vi "Prioridade_variaveis_server.vi"(8 "dados_entrada_vindo_client":T1, 11 "padrao_TAGS_prioridade_client":T5) -> (0 "dados_entrada_para_clp_priorizado":T1)   [LabVIEW 2019]
uses:
  padrao_TAGS_prioridades_client.ctl
  padrao_todos_os_dados_SAIDA.ctl
  padrao_UCM.004.EEL.0300_SAIDA.ctl
  padrao_UCM.004.EEL.0200_SAIDA.ctl
  padrao_INTERNO.ctl
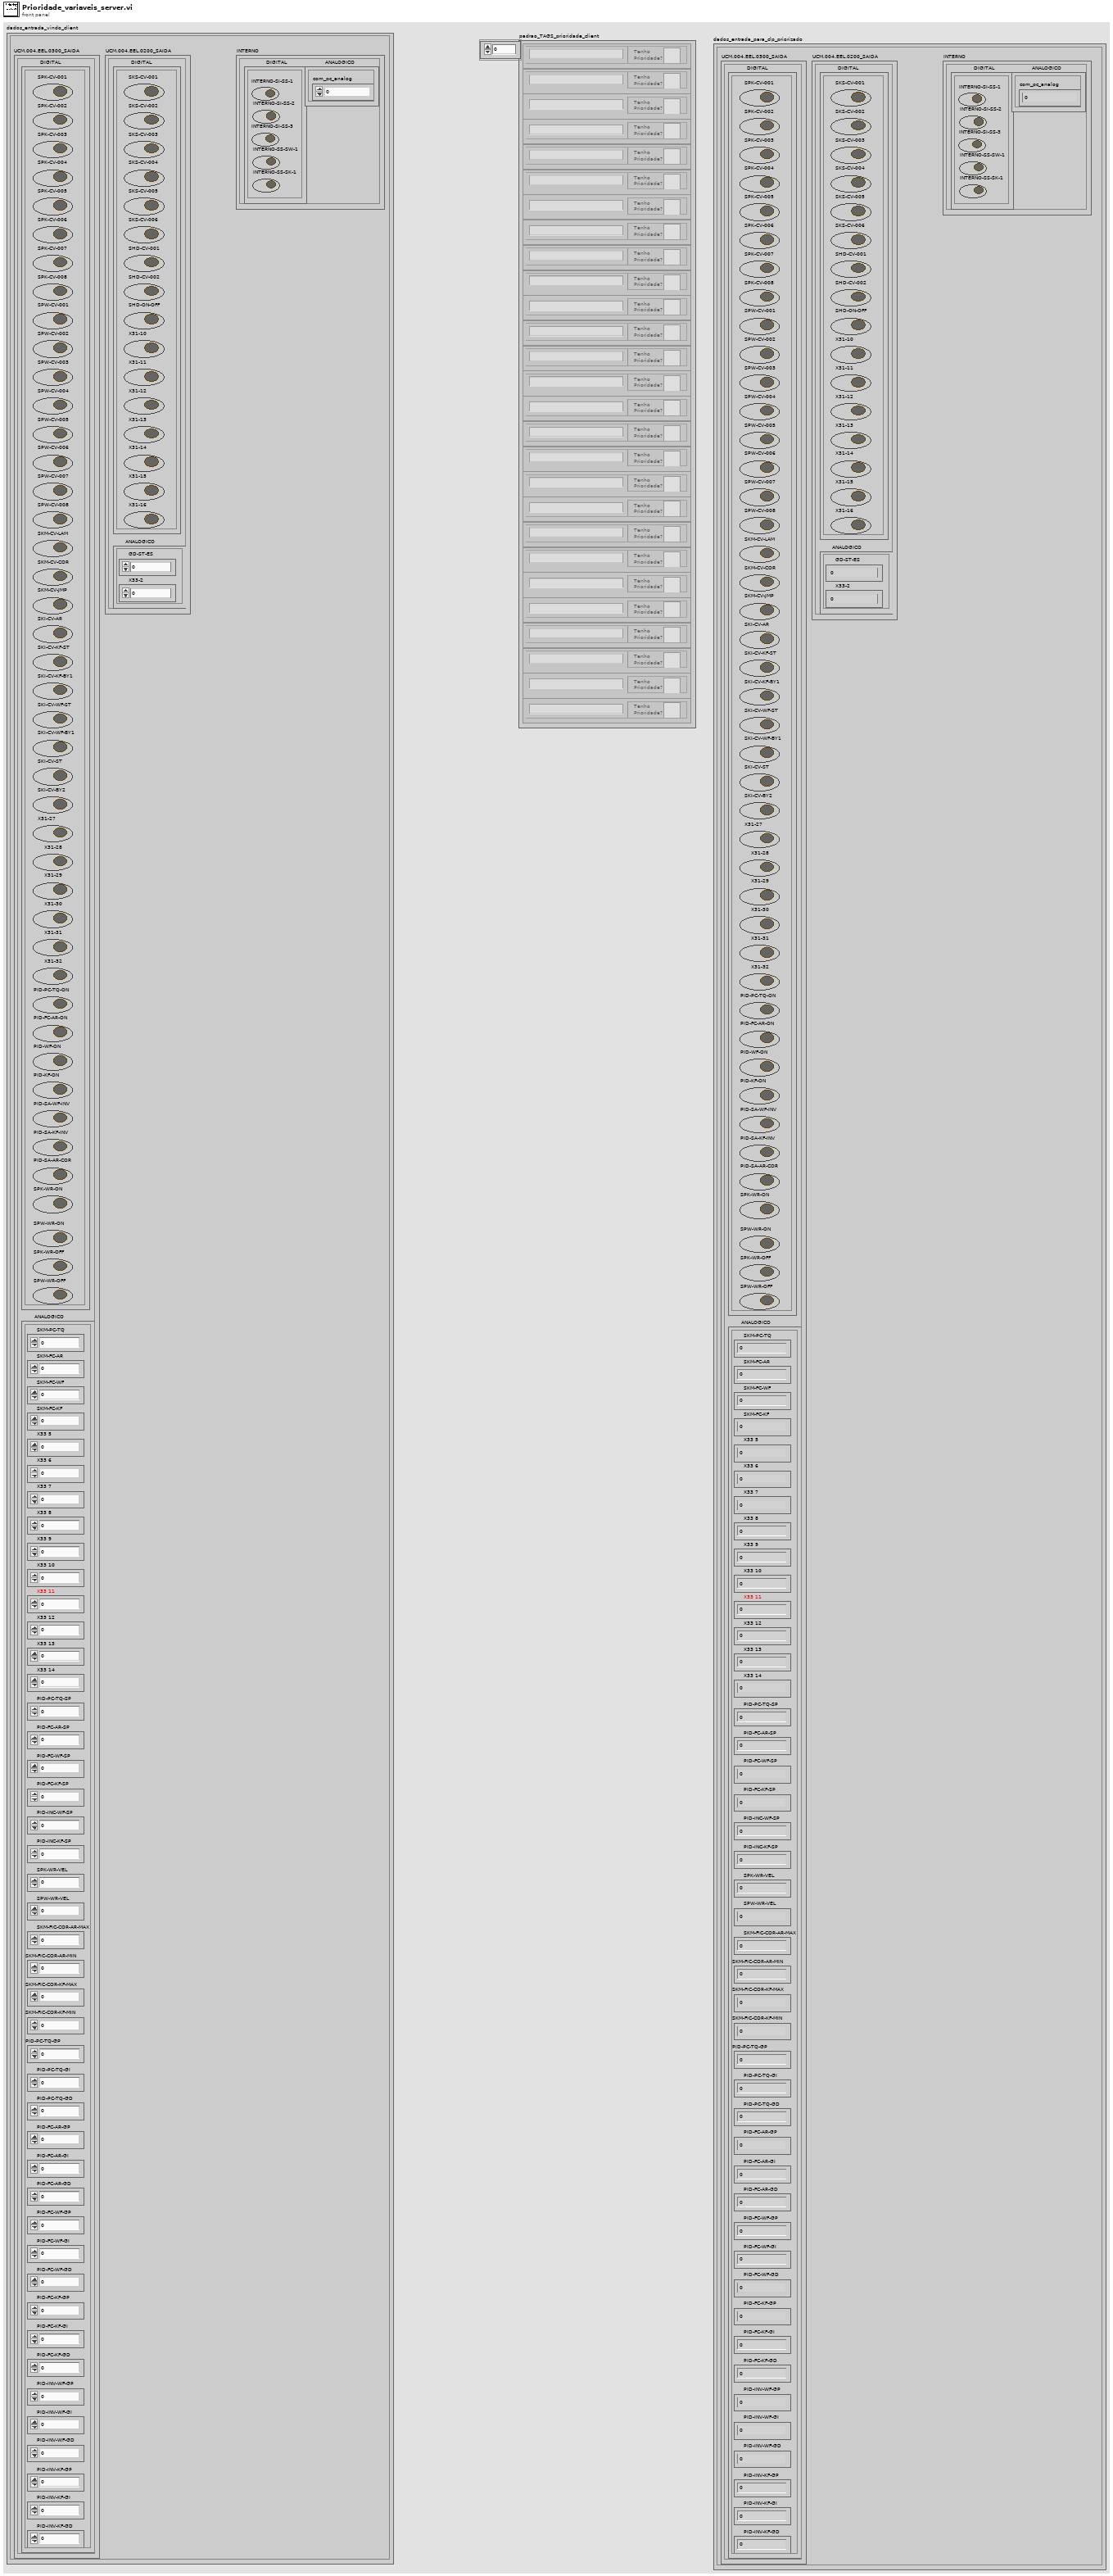
[diagram p1: front panel]
types:
  T1 = typedef "padrao_todos_os_dados_SAIDA.ctl" = cluster{"UCM.004.EEL.0300_SAIDA":T2, "UCM.004.EEL.0200_SAIDA":T3, "INTERNO":T4}
  T2 = typedef "padrao_UCM.004.EEL.0300_SAIDA.ctl" = cluster{"DIGITAL":cluster{"SPK-CV-001":bool, "SPK-CV-002":bool, "SPK-CV-003":bool, "SPK-CV-004":bool, "SPK-CV-005":bool, "SPK-CV-006":bool, "SPK-CV-007":bool, "SPK-CV-008":bool, "SPW-CV-001":bool, "SPW-CV-002":bool, "SPW-CV-003":bool, "SPW-CV-004":bool, "SPW-CV-005":bool, "SPW-CV-006":bool, "SPW-CV-007":bool, "SPW-CV-008":bool, "SKM-CV-LAM":bool, "SKM-CV-COR":bool, "SKM-CV-JMP":bool, "SKI-CV-AR":bool, "SKI-CV-KF-ST":bool, "SKI-CV-KF-BY1":bool, "SKI-CV-WF-ST":bool, "SKI-CV-WF-BY1":bool, "SKI-CV-ST":bool, "SKI-CV-BY2":bool, "X31-27":bool, "X31-28":bool, "X31-29":bool, "X31-30":bool, "X31-31":bool, "X31-32":bool, "PID-PC-TQ-ON":bool, "PID-FC-AR-ON":bool, "PID-WF-ON":bool, "PID-KF-ON":bool, "PID-SA-WF-INV":bool, "PID-SA-KF-INV":bool, "PID-SA-AR-COR":bool, "SPK-WR-ON":bool, "SPW-WR-ON":bool, "SPK-WR-OFF":bool, "SPW-WR-OFF":bool}, "ANALOGICO":cluster{"SKM-PC-TQ":i16, "SKM-FC-AR":i16, "SKM-FC-WF":i16, "SKM-FC-KF":i16, "X33 5":i16, "X33 6":i16, "X33 7":i16, "X33 8":i16, "X33 9":i16, "X33 10":i16, "X33 11":i16, "X33 12":i16, "X33 13":i16, "X33 14":i16, "PID-PC-TQ-SP":i16, "PID-FC-AR-SP":i16, "PID-FC-WF-SP":i16, "PID-FC-KF-SP":i16, "PID-INC-WF-SP":i16, "PID-INC-KF-SP":i16, "SPK-WR-VEL":i32, "SPW-WR-VEL":i32, "SKM-FIC-COR-AR-MAX":dbl, "SKM-FIC-COR-AR-MIN":dbl, "SKM-FIC-COR-KF-MAX":dbl, "SKM-FIC-COR-KF-MIN":dbl, "PID-PC-TQ-GP":dbl, "PID-PC-TQ-GI":dbl, "PID-PC-TQ-GD":dbl, "PID-FC-AR-GP":dbl, "PID-FC-AR-GI":dbl, "PID-FC-AR-GD":dbl, "PID-FC-WF-GP":dbl, "PID-FC-WF-GI":dbl, "PID-FC-WF-GD":dbl, "PID-FC-KF-GP":dbl, "PID-FC-KF-GI":dbl, "PID-FC-KF-GD":dbl, "PID-INV-WF-GP":dbl, "PID-INV-WF-GI":dbl, "PID-INV-WF-GD":dbl, "PID-INV-KF-GP":dbl, "PID-INV-KF-GI":dbl, "PID-INV-KF-GD":dbl}}
  T3 = typedef "padrao_UCM.004.EEL.0200_SAIDA.ctl" = cluster{"DIGITAL":cluster{"SKS-CV-001":bool, "SKS-CV-002":bool, "SKS-CV-003":bool, "SKS-CV-004":bool, "SKS-CV-005":bool, "SKS-CV-006":bool, "SHD-CV-001":bool, "SHD-CV-002":bool, "SHD-ON-OFF":bool, "X31-10":bool, "X31-11":bool, "X31-12":bool, "X31-13":bool, "X31-14":bool, "X31-15":bool, "X31-16":bool}, "ANALOGICO":cluster{"GD-ST-ES":i16, "X33-2":i16}}
  T4 = typedef "padrao_INTERNO.ctl" = cluster{"DIGITAL":cluster{"INTERNO-SI-SS-1":bool, "INTERNO-SI-SS-2":bool, "INTERNO-SI-SS-3":bool, "INTERNO-SS-SW-1":bool, "INTERNO-SS-SK-1":bool}, "ANALOGICO":cluster{"com_pc_analog":dbl}}
  T5 = typedef "padrao_TAGS_prioridades_client.ctl" = cluster{"TAG":string, "Tenho\nPrioridade?":bool}[]
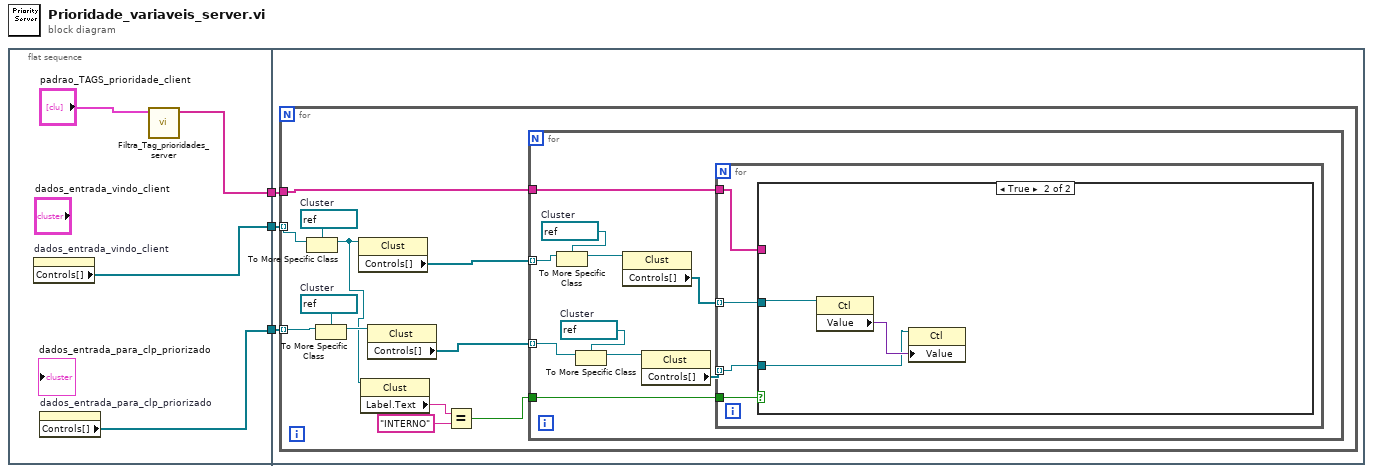
[diagram p0: block diagram]
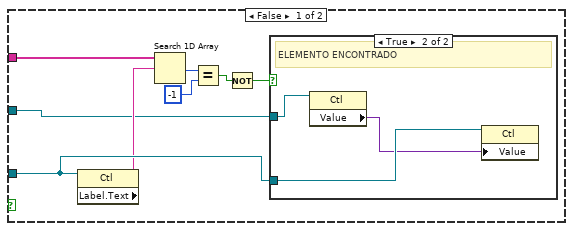
[diagram p2: hidden frame]
diagram:
  n1 = flat-sequence {
    tunnel: [w7] -> w3
    tunnel: [w5] -> w2
    tunnel: [w4] -> w1
    tunnel: w3 -> [w10]
    tunnel: w2 -> [w9]
    tunnel: w1 -> [w8]
    frame #0 {
      n2 = property on="dados_entrada_vindo_client" class="Clust (strict)"() -> ("Controls[]"=w4:refnum<vi>[])  [unwired: 2 in, 2 out]
      n3 = property on="dados_entrada_para_clp_priorizado" class="Clust (strict)"() -> ("Controls[]"=w7:refnum<vi>[])  [unwired: 2 in, 2 out]
      n4 = call "Filtra_Tag_prioridades_server.vi"("padrao_TAGS_prioridade_client"="padrao_TAGS_prioridade_client") -> ("TAGs prioridade"=w5:string[])  [unwired: 10 in]
    }
    frame #1 {
      n5 = for {
        tunnel: w10 -> [w19] mode=indexing
        tunnel: w9 -> [w18]
        tunnel: w8 -> [w16] mode=indexing
        w17 = refnum<vi> refnum  # Cluster
        w22 = refnum<vi> refnum  # Cluster
        n6 = To More Specific Class(target class=w17, reference=w16) -> (specific class reference=w14:refnum<vi>)  [unwired: 1 in, 1 out]
        n7 = To More Specific Class(target class=w22, reference=w19) -> (specific class reference=w20:refnum<vi>)  [unwired: 1 in, 1 out]
        n8 = property on="Property Node" class="Clust"(reference=w14) -> ("Controls[]"=w15:refnum<vi>[])  [unwired: 1 in, 2 out]
        n9 = property class="Clust"(reference=w14) -> ("Label.Text"=w13:string)  [unwired: 1 in, 2 out]
        n10 = property on="Property Node" class="Clust"(reference=w20) -> ("Controls[]"=w21:refnum<vi>[])  [unwired: 1 in, 2 out]
        n11 = Equal?(x=w13, y="INTERNO") -> (x = y?=w11:bool)
        n12 = for {
          tunnel: w21 -> [w31] mode=indexing
          tunnel: w18 -> [w28]
          tunnel: w15 -> [w25] mode=indexing
          tunnel: w11 -> [w23]
          w27 = refnum<vi> refnum  # Cluster
          w30 = refnum<vi> refnum  # Cluster
          n13 = To More Specific Class(target class=w27, reference=w25) -> (specific class reference=w26:refnum<vi>)  [unwired: 1 in, 1 out]
          n14 = To More Specific Class(target class=w30, reference=w31) -> (specific class reference=w32:refnum<vi>)  [unwired: 1 in, 1 out]
          n15 = property on="Property Node" class="Clust"(reference=w26) -> ("Controls[]"=w24:refnum<vi>[])  [unwired: 1 in, 2 out]
          n16 = property on="Property Node" class="Clust"(reference=w32) -> ("Controls[]"=w29:refnum<vi>[])  [unwired: 1 in, 2 out]
          n17 = for {
            tunnel: w29 -> [w36] mode=indexing
            tunnel: w28 -> [w35]
            tunnel: w24 -> [w34] mode=indexing
            tunnel: w23 -> [w33]
            n18 = case shown="True" w33 {
              tunnel: w36 -> [w44 w48]
              tunnel: w35 -> [w43 _]
              tunnel: w34 -> [w37 w49]
              frame False {
                n19 = property class="Ctl"(reference=w44) -> ("Label.Text"=w42:string)  [unwired: 1 in, 2 out]
                n20 = Search 1D Array(1D array=w43, element=w42) -> (index of element=w41:i32)  [unwired: 1 in]
                n21 = Equal?(x=w41, y=-1) -> (x = y?=w39:bool)
                n22 = Not(x=w39) -> (.not. x?=w38:bool)
                n23 = case shown="True" w38 {
                  tunnel: w44 -> [_ w47]
                  tunnel: w37 -> [_ w46]
                  frame False {
                    # "False: ELEMENTO NAO ENCONTRADO"
                  }
                  frame True {
                    # "ELEMENTO ENCONTRADO"
                    n24 = property class="Ctl"(reference=w46) -> ("Value"=w45:variant)  [unwired: 1 in, 2 out]
                    n25 = property class="Ctl"(reference=w47, "Value"=w45) -> ()  [unwired: 1 in, 2 out]
                  }
                }
              }
              frame True {
                n26 = property class="Ctl"(reference=w49) -> ("Value"=w50:variant)  [unwired: 1 in, 2 out]
                n27 = property class="Ctl"(reference=w48, "Value"=w50) -> ()  [unwired: 1 in, 2 out]
              }
            }
          }
        }
      }
    }
  }
